vi "KorrekturfaktorDin70020 (SubVI).vi"(10 "Lufttemperatur [°C]":dbl, 11 "Luftdruck [mbar]":dbl=1013.45) -> (3 "Numerisch":dbl)   [LabVIEW 2014]
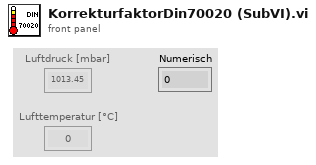
[diagram p1: front panel]
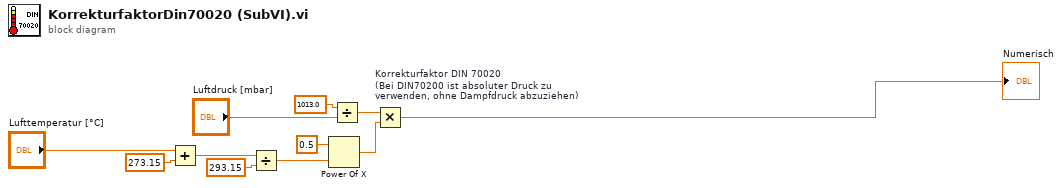
[diagram p0: block diagram]
diagram:
  n1 = Add(x="Lufttemperatur [°C]", y=273.15) -> (x+y=w4:dbl)
  n2 = Divide ("M_Welle [Nm]")(x=w4, y=293.15) -> (x/y=w6:dbl)
  n3 = Power Of X(1:w6, 2:0.5) -> (0:w9:dbl)
  n4 = Divide ("M_Welle [Nm]")(x=1013.0, y="Luftdruck [mbar]") -> (x/y=w8:dbl)
  n5 = Multiply "Korrekturfaktor DIN 70020 \n(Bei DIN70200 ist absoluter Druck zu verwenden, ohne Dampfdruck abzuziehen)"(x=w8, y=w9) -> (x*y=→"Numerisch":dbl)
